vi "enumerateStaticDependencies.vi"(8 "error in (no error)":errorcluster, 11 "Instrument":refnum<class "Instrument.lvclass">) -> (0 "error out":errorcluster, 2 "Static Dependencies":refnum<class "Dependency.lvclass">[](array[class]), 3 "Instrument out":refnum<class "Instrument.lvclass">)   [LabVIEW 2020, in "Instrument.lvclass"]
doc: "JKI State Machine Objects (SMO) 1.1.0.20\nJKI - JKI\nCopyright (c) 2016, JKI"
uses:
  Instrument.lvclass
  <vilib>/JKI/JKI SMO/Dependency/Dependency.lvclass
  Typedefs/Dependencies--Cluster.ctl
  <vilib>/JKI/JKI SMO/SMO/SMO.lvclass
panel:
  # "For instructions on how to use the JKI State Machine Objects, examples and video tutorials, visit:\nhttp://jki.net/state-machine-objects/\n\nJKI State Machine Objects™\nhttp://jki.net/state-machine-objects/\nCopyright (C) 2005-2015, JKI <info@jki.net>\nALL RIGHTS RESERVED"
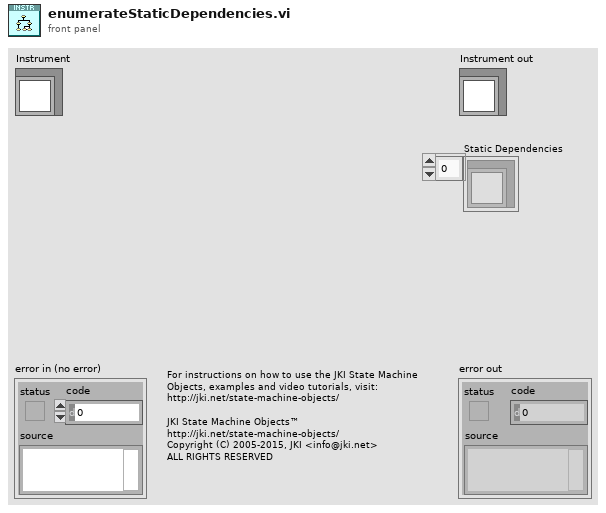
[diagram p1: front panel]
types:
  T1 = typedef "Instrument.lvclass/Dependencies--Cluster.ctl" = cluster{"Dep1":refnum<class "SMO.lvclass">, "Dep2":refnum<class "SMO.lvclass">}
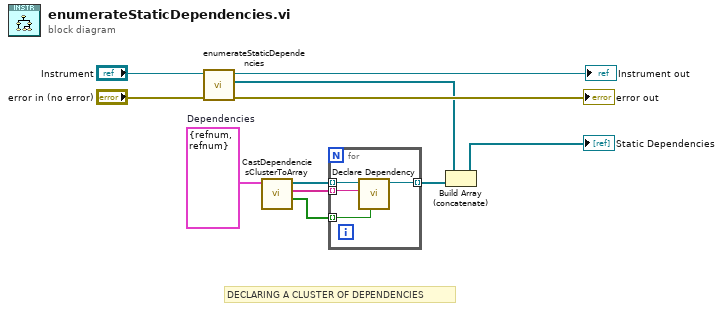
[diagram p0: block diagram]
diagram:
  w1 = T1 {"Dep1"=refnum, "Dep2"=refnum}  # Dependencies
  # "DECLARING A CLUSTER OF DEPENDENCIES"
  n1 = call-parent "enumerateStaticDependencies.vi"("error in (no error)"="error in (no error)", "SMO"="Instrument") -> ("error out"=→"error out":errorcluster, "Static Dependencies"=w2:refnum<class "Dependency.lvclass">[], "SMO out"=→"Instrument out":refnum<class "Instrument.lvclass">)  [unwired: 7 in]
  n2 = call <vilib>:"CastDependenciesClusterToArray.vi"("Dependencies Cluster"=w1) -> ("Shared Resources"=w3:bool[], "Dependencies Names"=w4:string[], "Dependencies Array"=w5:refnum<class "SMO.lvclass">[])  [unwired: 8 in]
  n3 = for {
    tunnel: [w15] -> w6 mode=indexing
    tunnel: w5 -> [w14] mode=indexing
    tunnel: w4 -> [w13] mode=indexing
    tunnel: w3 -> [w12] mode=indexing
    n4 = call <vilib>:"Declare Dependency.vi"("Shared Resource (F)"=w12, "Name"=w13, "Type"=w14) -> ("Dependency out"=w15:refnum<class "Dependency.lvclass">)  [unwired: 7 in, 1 out]
  }
  n5 = Build Array (concatenate)(w2, w6) -> (→"Static Dependencies":refnum<class "Dependency.lvclass">[])
